vi "niDTS Comm String Set Parameters Telnet.vi"(0 "Comm String Handle":T3, 5 "IP Address":string="192.168.1.200", 7 "Port Parameters Telnet":T2={"Bytes to Read"=1000, "Line Separator"="\n", "Port Timeout (ms)"=5000, "Read Mode"=enum."normal", "Write Mode"=enum."normal", "Remote Port"=23}, 9 "CLI Login":T1, 11 "error in (no error)":errorcluster) -> (4 "Comm String Handle Out":T3, 15 "error out":errorcluster)   [LabVIEW 2015, in "niDTS CommLib.lvlib"]
doc: "This sends the Command concatenated with the Args over the String Interface.\n\nInputs:\n* Command (Required): This is the command to be sent.\n* Args (Optional): Any arguments to be concatenated with the command.\n\nOutputs:\n* Response: Any data returned from the interface. Note that no data wil be returned if the flag Read Enabled is set to FALSE."
uses:
  niDTS CommLib.lvlib
  Includes/niDTS Comm String INC Handle.ctl
  Objects/String_class/niDTS Comm String.lvclass
  Includes/niDTS Comm INC Telnet Port Parameters.ctl
  Includes/niDTS Comm INC CLI Login.ctl
  Includes/niDTS Comm Telnet INC Handle.ctl
  Objects/Telnet_class/niDTS Comm Telnet.lvclass
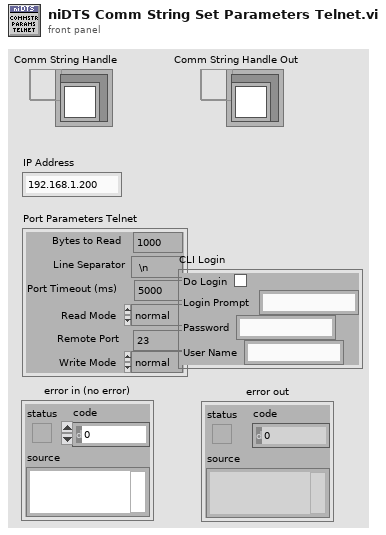
[diagram p1: front panel]
types:
  T1 = typedef "niDTS CommLib.lvlib/niDTS Comm INC CLI Login.ctl" = cluster{"Do Login":bool, "Login Prompt":string, "Password":string, "User Name":string}
  T2 = typedef "niDTS CommLib.lvlib/niDTS Comm INC Telnet Port Parameters.ctl" = cluster{"Bytes to Read":i32, "Line Separator":string, "Port Timeout (ms)":i32, "Read Mode":enum16{"normal", "line", "buffered"}, "Write Mode":enum16{"normal", "line", "buffered"}, "Remote Port":u16}
  T3 = typedef "niDTS CommLib.lvlib/niDTS Comm String INC Handle.ctl" = refnum<data-value>
  T4 = typedef "niDTS CommLib.lvlib/niDTS Comm Telnet INC Handle.ctl" = refnum<data-value>
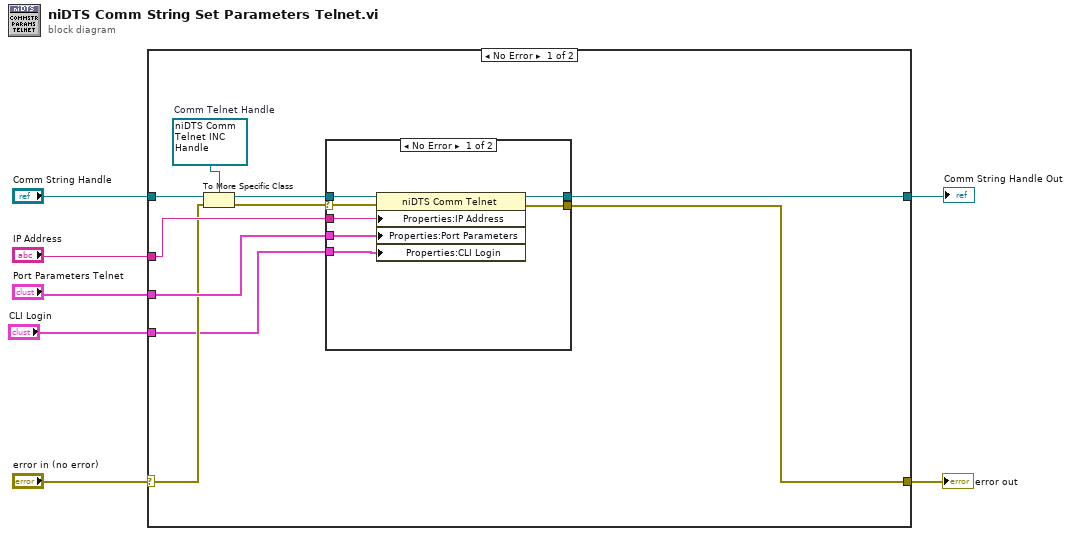
[diagram p0: block diagram]
diagram:
  n1 = case shown="No Error" "error in (no error)" {
    selector: "error in (no error)" -> [w10 w28]
    tunnel: [w9 w28] -> w7
    tunnel: "Comm String Handle" -> [w17 w27]
    tunnel: [w11 w27] -> w5
    tunnel: "IP Address" -> [w13 _]
    tunnel: "Port Parameters Telnet" -> [w12 _]
    tunnel: "CLI Login" -> [w8 _]
    frame No Error {
      w16 = T4 refnum  # Comm Telnet Handle
      n2 = To More Specific Class(target class=w16, reference=w17, error in=w10) -> (specific class reference=w14:T4, error out=w15:errorcluster)
      n3 = case shown="No Error" w15 {
        selector: w15 -> [w23 w25]
        tunnel: w14 -> [w24 w26]
        tunnel: w13 -> [w22 _]
        tunnel: w12 -> [w21 _]
        tunnel: [w20 w26] -> w11
        tunnel: [w19 w25] -> w9
        tunnel: w8 -> [w18 _]
        frame No Error {
          n4 = property class="niDTS Comm Telnet"(reference=w24, error in=w23, "Properties:IP Address"=w22, "Properties:Port Parameters"=w21, "Properties:CLI Login"=w18) -> (reference out=w20:T4, error out=w19:errorcluster)
        }
        frame Error {
        }
      }
    }
    frame Error {
    }
  }
  "error out" <- w7
  "Comm String Handle Out" <- w5
